vi "SetSweepParameters.vi"(8 "error in (no error)":errorcluster, 9 "Points":i32, 10 "Sweep Time (ms)":dbl format="%#_13g", 11 "SpectrumAnalyzer in":refnum<class "SpectrumAnalyzer.lvclass">) -> (0 "error out":errorcluster, 3 "SpectrumAnalyzer out":refnum<class "SpectrumAnalyzer.lvclass">)   [LabVIEW 2023, in "SpectrumAnalyzerInterface.lvlib" / "SpectrumAnalyzer.lvclass"]
uses:
  SpectrumAnalyzer.lvclass
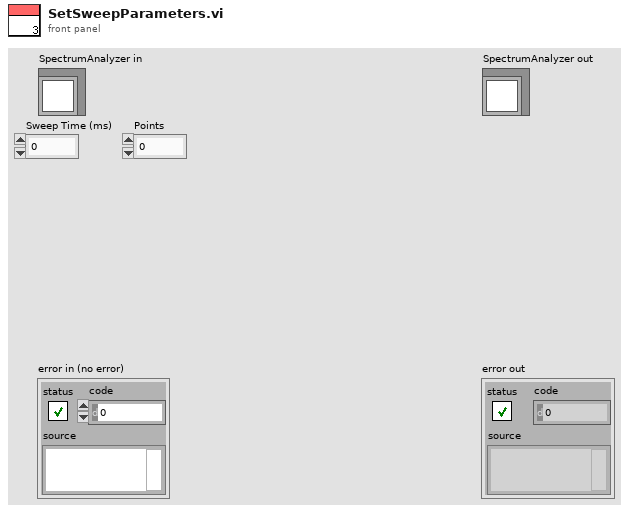
[diagram p1: front panel]
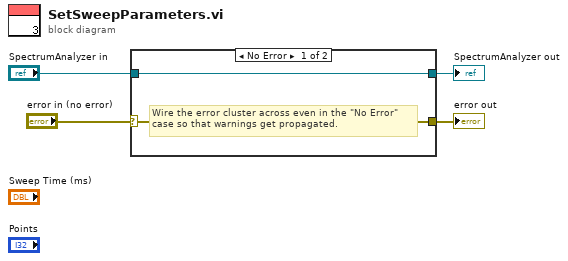
[diagram p0: block diagram]
diagram:
  n1 = case shown="No Error" "error in (no error)" {
    selector: "error in (no error)" -> [w5 w8]
    tunnel: [w5 w8] -> w3
    tunnel: [w6 w7] -> w1
    tunnel: "SpectrumAnalyzer in" -> [w6 w7]
    frame No Error {
      # "Wire the error cluster across even in the \"No Error\"\ncase so that warnings get propagated."
    }
    frame Error {
    }
  }
  "error out" <- w3
  "SpectrumAnalyzer out" <- w1
